vi "Julian_Date_2.vi"() -> (2 "Julian Date":dbl format="%.4g")   [LabVIEW 2012]
panel:
  out "current time":timestamp
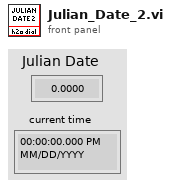
[diagram p1: front panel]
types:
  T1 = typedef "LVDateTimeRec.ctl" = cluster{"fractional second":dbl, "second":i32, "minute":i32, "hour":i32, "day of month":i32, "month":i32, "year":i32, "day of week":i32, "day of year":i32, "DST":i32}
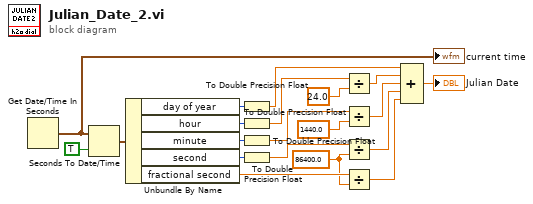
[diagram p0: block diagram]
diagram:
  w1 = 86400.0 ("y")
  n1 = Get Date/Time In Seconds() -> (seconds since 1Jan1904=w20:timestamp)
  "current time" <- w20
  n2 = Seconds To Date/Time(time stamp (now)=w20, to UTC (F)=TRUE) -> (date time rec=w18:T1)
  n3 = Unbundle By Name(w18) -> ("day of year"=w17:i32, "hour"=w16:i32, "minute"=w15:i32, "second"=w14:i32, "fractional second"=w3:dbl)
  n4 = To Double Precision Float(number=w17) -> (double precision float=w8:dbl)
  n5 = To Double Precision Float(number=w16) -> (double precision float=w12:dbl)
  n6 = To Double Precision Float(number=w15) -> (double precision float=w10:dbl)
  n7 = To Double Precision Float(number=w14) -> (double precision float=w9:dbl)
  n8 = Divide(x=w12, y=24.0) -> (x/y=w7:dbl)
  n9 = Divide(x=w10, y=1440.0) -> (x/y=w6:dbl)
  n10 = Divide(x=w9, y=w1) -> (x/y=w5:dbl)
  n11 = Divide(x=w3, y=w1) -> (x/y=w2:dbl)
  n12 = Compound Arithmetic op=ADD(w8, w7, w6, w5, w2) -> (→"Julian Date":dbl)
